vi "stopTempController.vi"(8 "error in (no error)":errorcluster, 9 "releaseWhenReady":bool, 11 "CameraManager in":refnum<class "CameraManager.lvclass">) -> (0 "error out":errorcluster, 3 "CameraManager out":refnum<class "CameraManager.lvclass">)   [LabVIEW 2011, in "iManagement.lvlib" / "CameraManager.lvclass"]
doc: "Closes the temperature controller of the camera.\nNormally it will wait for it to warm up to a specific safe \ntemperature before shutting it down."
uses:
  CameraManager.lvclass
  CameraManager.lvclass/CameraManager.ctl
  Hal/Channels/Camera/CameraController.lvclass
  Hal/Channels/Camera/CameraEventsManager/CameraEventsManger.lvclass
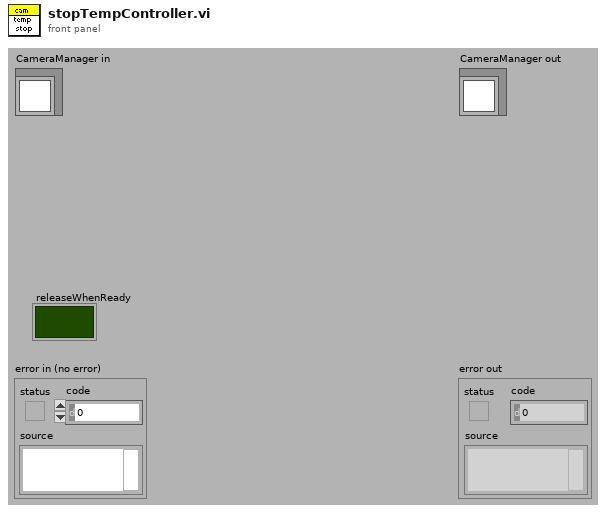
[diagram p1: front panel]
types:
  T1 = cluster{"newSetPointEvent":refnum<user-event>, "stopCoolingEvent":refnum<user-event>}
  T2 = cluster{"closeEvent":refnum<user-event>, "temperatureUpdateEvent":refnum<user-event>, "displayErrorEvent":refnum<user-event>, "setPointUpdateEvent":refnum<user-event>}
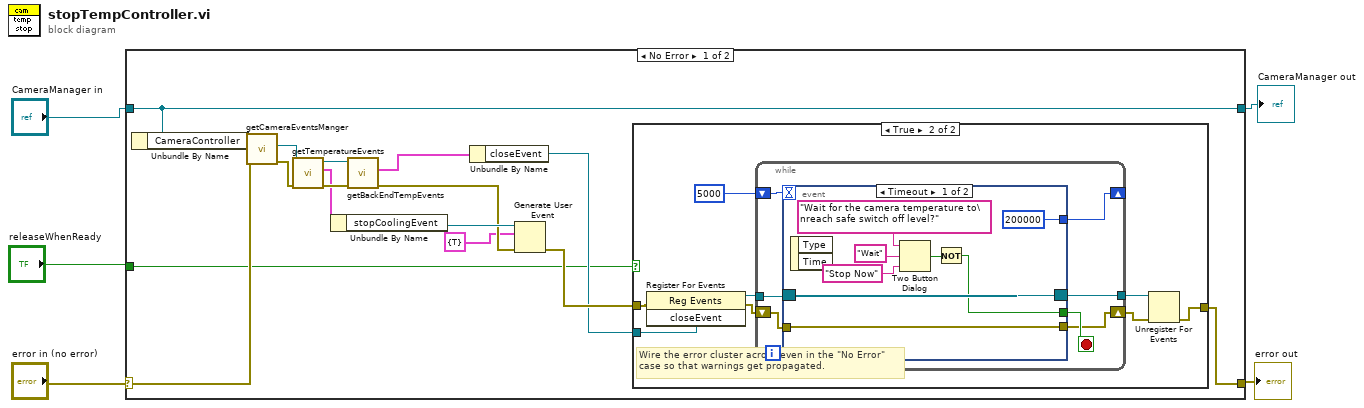
[diagram p0: block diagram]
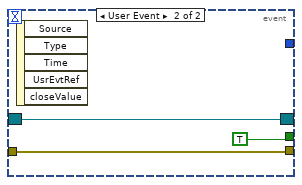
[diagram p3: hidden frame]
diagram:
  # "Wire the error cluster across even in the \"No Error\"\ncase so that warnings get propagated."
  n1 = case shown="No Error" "error in (no error)" {
    selector: "error in (no error)" -> [w19 w50]
    tunnel: [w9 w50] -> w1
    tunnel: [w21 w49] -> w2
    tunnel: "CameraManager in" -> [w21 w49]
    tunnel: "releaseWhenReady" -> [w6 _]
    frame No Error {
      n2 = Unbundle By Name(w21) -> ("CameraController"=w20:refnum<class "CameraController.lvclass">)
      n3 = call-dynamic "getCameraEventsManger.vi"("error in (no error)"=w19, "CameraController.lvclass in"=w20) -> ("error out"=w13:errorcluster, "Hardware:Channels.lvlib:CameraEventsManger.lvclass"=w18:refnum<class "CameraEventsManger.lvclass">)  [unwired: 7 in, 1 out]
      n4 = call-dynamic "getTemperatureEvents.vi"("error in (no error)"=w13, "CameraEventsManger.lvclass in"=w18) -> ("error out"=w17:errorcluster, "temperatureEvents"=w8:T1, "CameraEventsManger.lvclass out"=w16:refnum<class "CameraEventsManger.lvclass">)  [unwired: 7 in]
      n5 = Unbundle By Name(w8) -> ("stopCoolingEvent"=w15:refnum<user-event>)
      n6 = call-dynamic "getBackEndTempEvents.vi"("error in (no error)"=w17, "CameraEventsManger.lvclass in"=w16) -> ("error out"=w14:errorcluster, "backEndTempEvents"=w12:T2)  [unwired: 7 in, 1 out]
      n7 = Unbundle By Name(w12) -> ("closeEvent"=w10:refnum<user-event>)
      n8 = Generate User Event(user event=w15, event data cluster=cluster{"stopValue":bool} {"stopValue"=TRUE} ("event data"), error in=w14) -> (error out=w11:errorcluster)  [unwired: 1 out]
      n9 = case shown="True" w6 {
        tunnel: w11 -> [w22 w30]
        tunnel: w10 -> [_ w27]
        tunnel: [w22 w24] -> w9
        frame False {
        }
        frame True {
          n10 = register-events(error in=w30, w27) -> (reference out=w29:refnum<event-registration>, error out=w28:errorcluster)  [unwired: 1 in]
          n11 = while {
            tunnel: w29 -> [w37]
            shift-right: [w34] -> w25
            shift-left: w28 -> [w36]
            tunnel: [w33] -> w26
            shift-right: [w31] -> _
            shift-left: 5000 -> [w32]
            stop <- w35 stop-if-true
            n12 = event shown="[0] Timeout" {
              selector: w37 -> [w45 w48]
              dyn-events: [w45 w48] -> w33
              timeout: w32 -> [_ _]
              tunnel: w36 -> [w44 w46]
              tunnel: [w39 TRUE] -> w35
              tunnel: [w44 w46] -> w34
              tunnel: [200000 _] -> w31
              event Timeout {
                n13 = event-data() -> ()  [unwired: 1 in, 2 out]
                n14 = Two Button Dialog(message="Wait for the camera temperature to\nreach safe switch off level?", 1:"Stop Now", 2:"Wait") -> (T button?=w40:bool)
                n15 = Not(x=w40) -> (.not. x?=w39:bool)
              }
              event User Event {
                n16 = event-data() -> ()  [unwired: 1 in, 5 out]
              }
            }
          }
          n17 = Unregister For Events(event registration refnum=w26, error in=w25) -> (error out=w24:errorcluster)
        }
      }
    }
    frame Error {
    }
  }
  "error out" <- w1
  "CameraManager out" <- w2
